vi "Pre Launch Init.vi"(11 "Nested in":refnum<class "Binary counter.lvclass">) -> (0 "error out":errorcluster, 3 "Nested out":refnum<class "Binary counter.lvclass">)   [LabVIEW 2020, in "Binary counter.lvlib" / "Binary counter.lvclass"]
doc: "(<B>Filename</B>: Actor Framework.lvlib:Actor.lvclass:Pre Launch Init.vi)\n\nDefines behavior that occurs after the Launch Nested Actor method is invoked but before the actor's Actor Core method begins running.\n\nBy default, this method does nothing. A descendant class may override it to define behavior."
uses:
  Binary counter.lvclass
  Binary counter.lvclass/Binary counter.ctl
  <vilib>/ActorFramework/Actor/Actor.lvclass
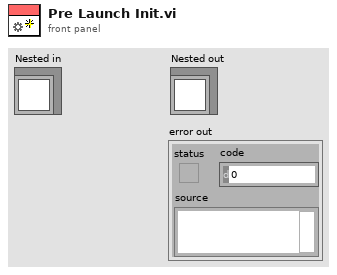
[diagram p1: front panel]
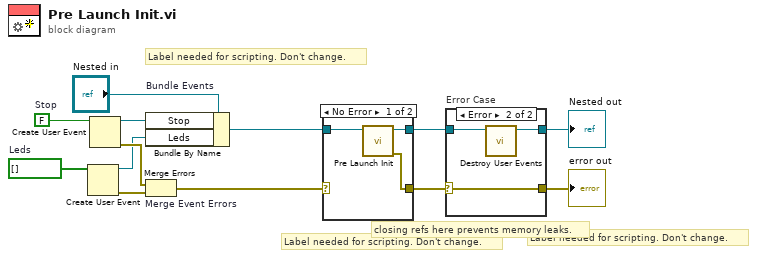
[diagram p0: block diagram]
diagram:
  w3 = bool[] []  # Leds
  w12 = FALSE  # Stop
  # "Label needed for scripting. Don't change."
  # "Label needed for scripting. Don't change."
  # "Label needed for scripting. Don't change."
  # "closing refs here prevents memory leaks."
  n1 = Create User Event(user event datatype=w3) -> (user event=w2:refnum<user-event>, error out=w1:errorcluster)  [unwired: 1 in]
  n2 = Create User Event(user event datatype=w12) -> (user event=w9:refnum<user-event>, error out=w11:errorcluster)  [unwired: 1 in]
  n3 = Bundle By Name "Bundle Events"(cluster="Nested in", "Stop"=w9, "Leds"=w2) -> (w6:refnum<class "Binary counter.lvclass">)
  n4 = Merge Errors "Merge Event Errors"(w11, w1) -> (w5:errorcluster)
  n5 = case shown="No Error" w5 {
    selector: w5 -> [_ w18]
    tunnel: [w16 w17] -> w7
    tunnel: w6 -> [w15 w17]
    tunnel: [w14 w18] -> w4
    frame No Error {
      n6 = call-parent "Pre Launch Init.vi"("Actor in"=w15) -> ("error out"=w14:errorcluster, "Actor out"=w16:refnum<class "Binary counter.lvclass">)  [unwired: 9 in]
    }
    frame Error {
    }
  }
  n7 = case "Error Case" shown="Error" w4 {
    selector: w4 -> [w19 w23]
    tunnel: w7 -> [w20 w22]
    tunnel: [w20 w21] -> w10
    tunnel: [w19 w23] -> w8
    frame No Error {
    }
    frame Error {
      n8 = call "Destroy User Events.vi"("UI Template in"=w22) -> ("UI Template out"=w21:refnum<class "Binary counter.lvclass">)  [unwired: 10 in]
    }
  }
  "error out" <- w8
  "Nested out" <- w10
